vi "digital input pointer to sequence text.vi"(11 "Digital Input":T1) -> (3 "String":string)   [LabVIEW 2018]
uses:
  type defs/Digital Input Pointer.ctl
  type defs/MCAS Digital Input Control_single nest.ctl
  type defs/misc digital input.ctl
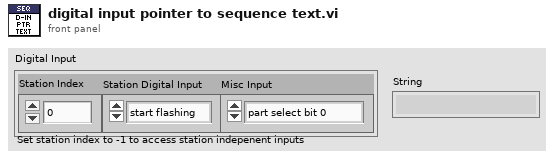
[diagram p1: front panel]
types:
  T1 = typedef "Digital Input Pointer.ctl" = cluster{"Station Digital Input":T2, "Station Index":i32, "Misc Input":T3}
  T2 = typedef "MCAS Digital Input Control_single nest.ctl" = enum16{"start flashing", "reject", "part present 1", "part present 2", "clamp opened", "clamp closed", "tool select bit 0", "tool select bit 1"}
  T3 = typedef "misc digital input.ctl" = enum16{"part select bit 0", "part select bit 1", "part select bit 2", "part select bit 3"}
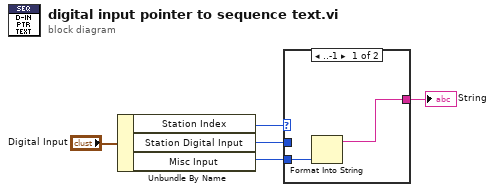
[diagram p0: block diagram]
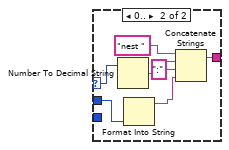
[diagram p2: hidden frame]
diagram:
  n1 = Unbundle By Name("Digital Input") -> ("Station Index"=w2:i32, "Station Digital Input"=w4:T2, "Misc Input"=w3:T3)
  n2 = case shown="..-1" w2 {
    selector: w2 -> [_ w12]
    tunnel: w3 -> [w7 _]
    tunnel: w4 -> [_ w14]
    tunnel: [w6 w10] -> w5
    frame ..-1 {
      n3 = Format Into String(w7) -> (resulting string=w6:string)  [unwired: 3 in, 1 out]
    }
    frame 0.. {
      n4 = Number To Decimal String(number=w12) -> (decimal integer string=w11:string)  [unwired: 1 in]
      n5 = Format Into String(w14) -> (resulting string=w8:string)  [unwired: 3 in, 1 out]
      n6 = Concatenate Strings("nest ", w11, ":" ("string"), w8) -> (w10:string)
    }
  }
  "String" <- w5
